vi "AOL Control.vi"() -> ()   [LabVIEW 2017]
uses:
  TypeDef/Frequency.ctl
  TypeDef/Amplitude.ctl
  TypeDef/AOL Mode.ctl
  Globals/FPGA Globals.vi
  <vilib>/DAQmx/create/channels.llb/DAQmx Create Channel (CO-Pulse Generation-Time).vi
panel:
  in  "DAQmx Digital Channel":tag="Dev1/ctr0"
  in  "Initial Delay(sec)":dbl=0.01 format="%.6f"
  in  "High Time(sec)":dbl=1e-05
  in  "Low Time(sec)":dbl=0.1
  in  "error in":errorcluster
  out "Select Device 2":i32=1 min=1 max=5 step=1
  out "Select Device 1":i32=1 min=1 max=5 step=1
  in  "Settings":bool
  in  "Refresh":bool
  in  "Save As":bool
  in  "Clear":bool
  in  "Run":bool
  in  "Load":bool
  in  "Stop":bool
  out "No of Packets":i32
  out "Packet Array":string[](array[string])
  in  "AOL Mode":T1=enum."Alignment"
  in  "Amplitude":T2={"Ch 1"=210, "Ch 2"=200, "Ch 3"=227, "Ch 4"=220, "Ch 5"=130, "Ch 6"=100, "Ch 7"=120, "Ch 8"=100}
  in  "Frequency (MHz)":T3={"Ch 1"=39, "Ch 2"=39, "Ch 3"=39, "Ch 4"=39, "Ch 5"=39, "Ch 6"=39, "Ch 7"=39, "Ch 8"=39}
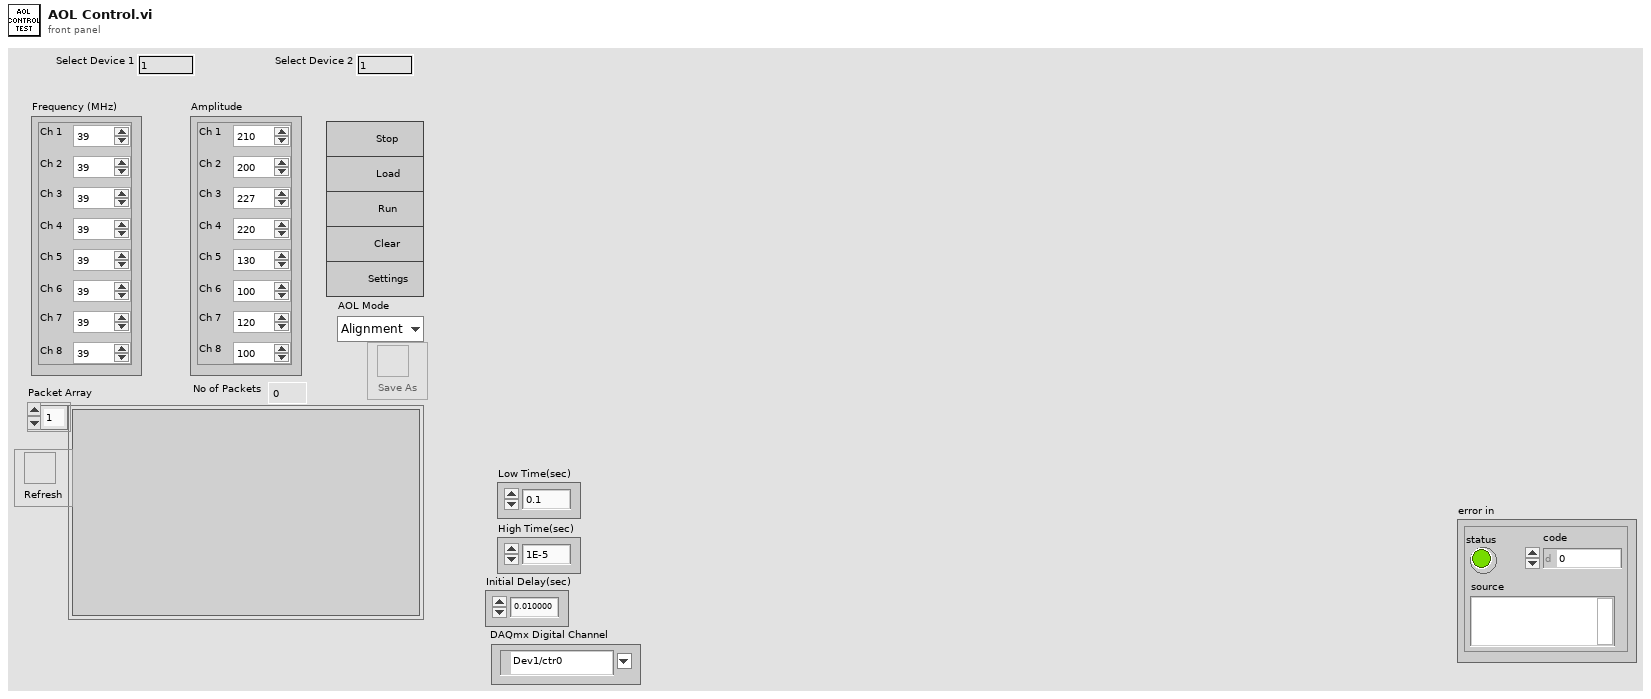
[diagram p1: front panel]
types:
  T1 = typedef "AOL Mode.ctl" = enum16{"Raster", "Structural", "Functional", "MiniScan", "Alignment"}
  T2 = typedef "Amplitude.ctl" = cluster{"Ch 1":u16, "Ch 2":u16, "Ch 3":u16, "Ch 4":u16, "Ch 5":u16, "Ch 6":u16, "Ch 7":u16, "Ch 8":u16}
  T3 = typedef "Frequency.ctl" = cluster{"Ch 1":u16, "Ch 2":u16, "Ch 3":u16, "Ch 4":u16, "Ch 5":u16, "Ch 6":u16, "Ch 7":u16, "Ch 8":u16}
  T4 = typedef "FPGA Settings.ctl" = cluster{"System Clock(MHz)":dbl, "FPGA MAC 1":string, "Port Number 1":i32, "Port Number 2":i32, "FPGA MAC 2":string}
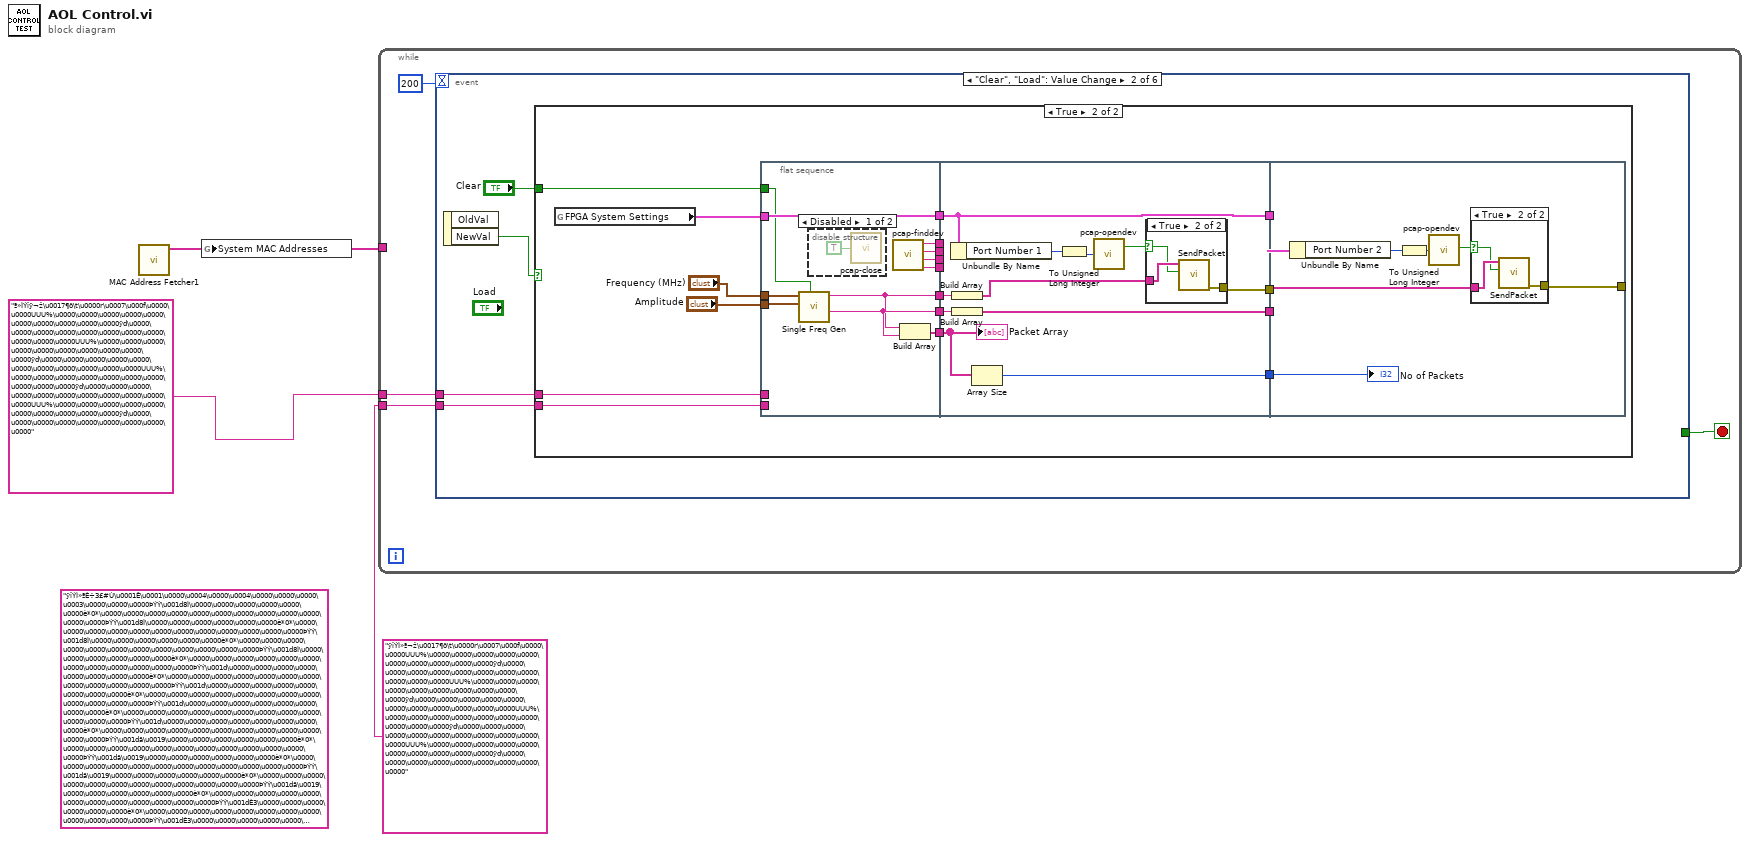
[diagram p0: block diagram]
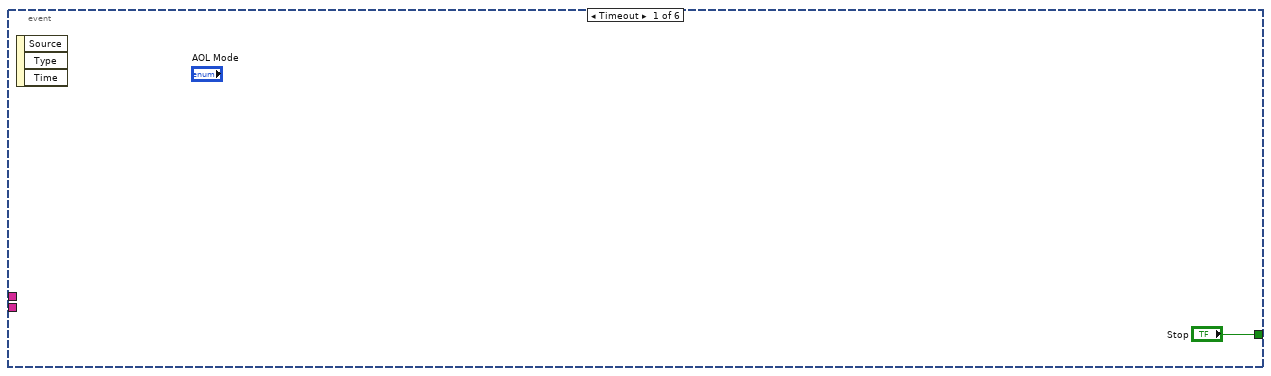
[diagram p2: hidden frame]
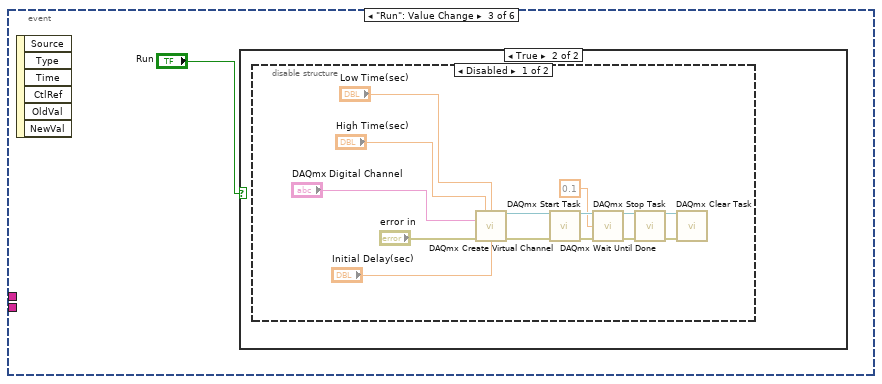
[diagram p7: hidden frame]
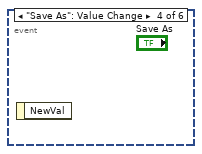
[diagram p10: hidden frame]
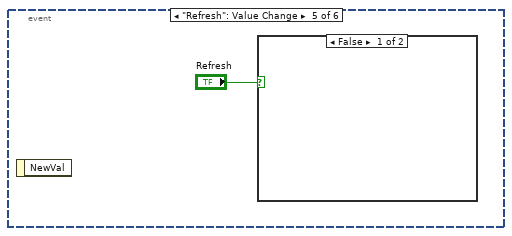
[diagram p11: hidden frame]
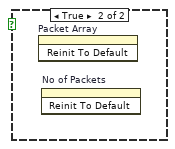
[diagram p12: hidden frame]
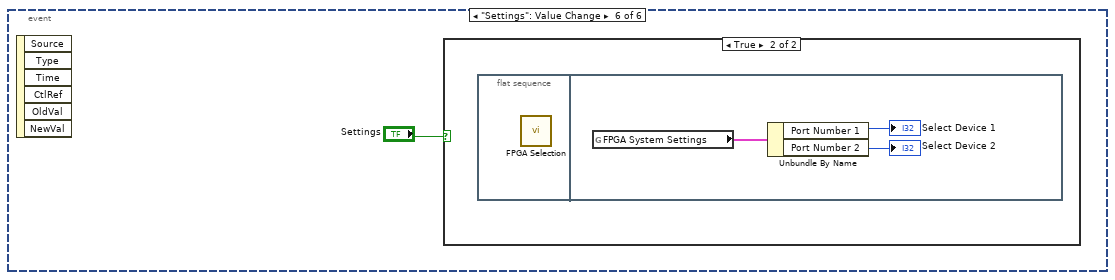
[diagram p13: hidden frame]
diagram:
  (unwired) "ÿîÝÌ»ªÈ÷3£#Ù\u0001Ê\u0001\u0000\u0004\u0000\u0004\u0000\u0000\u0000\u0003\u0000\u0000\u0000ÞÝÝ\u001d8Ì\u0000\u0000\u0000\u0000\u0000\u0000è*0*\u0000\u0000\u0000\u0000\u0000\u0000\u0000\u0000\u0000\u0000\u0000\u0000ÞÝÝ\u001d8Ì\u0000\u0000\u0000\u0000\u0000\u0000è*0*\u0000\u0000\u0000\u0000\u0000\u0000\u0000\u0000\u0000\u0000\u0000\u0000ÞÝÝ\u001d8Ì\u0000\u0000\u0000\u0000\u0000\u0000è*0*\u0000\u0000\u0000\u0000\u0000\u0000\u0000\u0000\u0000\u0000\u0000\u0000ÞÝÝ\u001d8Ì\u0000\u0000\u0000\u0000\u0000\u0000è*0*\u0000\u0000\u0000\u0000\u0000\u0000\u0000\u0000\u0000\u0000\u0000\u0000ÞÝÝ\u001d\u0000\u0000\u0000\u0000\u0000\u0000\u0000\u0000è*0*\u0000\u0000\u0000\u0000\u0000\u0000\u0000\u0000\u0000\u0000\u0000\u0000ÞÝÝ\u001d\u0000\u0000\u0000\u0000\u0000\u0000\u0000\u0000è*0*\u0000\u0000\u0000\u0000\u0000\u0000\u0000\u0000\u0000\u0000\u0000\u0000ÞÝÝ\u001d\u0000\u0000\u0000\u0000\u0000\u0000\u0000\u0000è*0*\u0000\u0000\u0000\u0000\u0000\u0000\u0000\u0000\u0000\u0000\u0000\u0000ÞÝÝ\u001d\u0000\u0000\u0000\u0000\u0000\u0000\u0000\u0000è*0*\u0000\u0000\u0000\u0000\u0000\u0000\u0000\u0000\u0000\u0000\u0000\u0000ÞÝÝ\u001dä\u0019\u0000\u0000\u0000\u0000\u0000\u0000è*0*\u0000\u0000\u0000\u0000\u0000\u0000\u0000\u0000\u0000\u0000\u0000\u0000ÞÝÝ\u001dä\u0019\u0000\u0000\u0000\u0000\u0000\u0000è*0*\u0000\u0000\u0000\u0000\u0000\u0000\u0000\u0000\u0000\u0000\u0000\u0000ÞÝÝ\u001dä\u0019\u0000\u0000\u0000\u0000\u0000\u0000è*0*\u0000\u0000\u0000\u0000\u0000\u0000\u0000\u0000\u0000\u0000\u0000\u0000ÞÝÝ\u001dä\u0019\u0000\u0000\u0000\u0000\u0000\u0000è*0*\u0000\u0000\u0000\u0000\u0000\u0000\u0000\u0000\u0000\u0000\u0000\u0000ÞÝÝ\u001dÈ3\u0000\u0000\u0000\u0000\u0000\u0000è*0*\u0000\u0000\u0000\u0000\u0000\u0000\u0000\u0000\u0000\u0000\u0000\u0000ÞÝÝ\u001dÈ3\u0000\u0000\u0000\u0000\u0000\u0000è*0*\u0000\u0000\u0000\u0000\u0000\u0000\u0000\u0000\u0000\u0000\u0000\u0000ÞÝÝ\u001dÈ3\u0000\u0000\u0000\u0000\u0000\u0000è*0*\u0000\u0000\u0000\u0000\u0000\u0000\u0000\u0000\u0000\u0000\u0000\u0000ÞÝÝ\u001dÈ3\u0000\u0000\u0000\u0000\u0000\u0000è*0*\u0000\u0000\u0000\u0000\u0000\u0000\u0000\u0000\u0000\u0000"
  n1 = call "MAC Address Fetcher1.vi"() -> ("MAC Addresses"=w3:string[])  [unwired: 9 in, 2 out]
  n2 = global write "FPGA Globals.vi" "System MAC Addresses"(w3) -> ()
  n3 = while {
    tunnel: w3 -> [_]
    tunnel: "ª»ÌÝîÿ¬ž\u0017¶ö\t\u0000r\u0007\u000f\u0000\u0000UUU%\u0000\u0000\u0000\u0000\u0000\u0000\u0000\u0000\u0000\u0000ÿd\u0000\u0000\u0000\u0000\u0000\u0000\u0000\u0000\u0000\u0000\u0000UUU%\u0000\u0000\u0000\u0000\u0000\u0000\u0000\u0000\u0000\u0000ÿd\u0000\u0000\u0000\u0000\u0000\u0000\u0000\u0000\u0000\u0000\u0000UUU%\u0000\u0000\u0000\u0000\u0000\u0000\u0000\u0000\u0000\u0000ÿd\u0000\u0000\u0000\u0000\u0000\u0000\u0000\u0000\u0000\u0000\u0000UUU%\u0000\u0000\u0000\u0000\u0000\u0000\u0000\u0000\u0000\u0000ÿd\u0000\u0000\u0000\u0000\u0000\u0000\u0000\u0000\u0000" ("String") -> [w5]
    tunnel: "ÿîÝÌ»ª¬ž\u0017¶ö\t\u0000r\u0007\u000f\u0000\u0000UUU%\u0000\u0000\u0000\u0000\u0000\u0000\u0000\u0000\u0000\u0000ÿd\u0000\u0000\u0000\u0000\u0000\u0000\u0000\u0000\u0000\u0000\u0000UUU%\u0000\u0000\u0000\u0000\u0000\u0000\u0000\u0000\u0000\u0000ÿd\u0000\u0000\u0000\u0000\u0000\u0000\u0000\u0000\u0000\u0000\u0000UUU%\u0000\u0000\u0000\u0000\u0000\u0000\u0000\u0000\u0000\u0000ÿd\u0000\u0000\u0000\u0000\u0000\u0000\u0000\u0000\u0000\u0000\u0000UUU%\u0000\u0000\u0000\u0000\u0000\u0000\u0000\u0000\u0000\u0000ÿd\u0000\u0000\u0000\u0000\u0000\u0000\u0000\u0000\u0000" ("String") -> [w4]
    stop <- w6 stop-if-true
    n4 = event shown="[1] \"Clear\", \"Load\": Value Change" {
      selector: _ -> [_ _ _ _ _ _]
      dyn-events: _ -> [_ _ _ _ _ _]
      timeout: 200 -> [_ _ _ _ _ _]
      tunnel: ["Stop" _ _ _ _ _] -> w6
      tunnel: w5 -> [_ w10 _ _ _ _]
      tunnel: w4 -> [_ w9 _ _ _ _]
      event Timeout {
        n5 = event-data() -> ()  [unwired: 1 in, 3 out]
      }
      event "Clear", "Load": Value Change {
        n6 = event-data() -> ("NewVal"=w12:bool)  [unwired: 1 in, 1 out]
        n7 = case shown="True" w12 {
          tunnel: "Clear" -> [_ w21]
          tunnel: w10 -> [_ w16]
          tunnel: w9 -> [_ w15]
          frame False {
          }
          frame True {
            n8 = global read "FPGA Globals.vi" "FPGA System Settings"() -> (w22:T4)
            n9 = flat-sequence {
              tunnel: "Amplitude" -> [w41]
              tunnel: "Frequency (MHz)" -> [w40]
              tunnel: [w39] -> w30
              tunnel: [w38] -> w29
              tunnel: w22 -> [w38]
              tunnel: w21 -> [w37]
              tunnel: [w36] -> w20
              tunnel: [w35] -> w19
              tunnel: [w34] -> w18
              tunnel: [w33] -> w17
              tunnel: w16 -> [_]
              tunnel: w15 -> [_]
              tunnel: [w31] -> w14
              tunnel: [w32] -> w13
              tunnel: [w52] -> w28
              tunnel: [w48] -> w27
              tunnel: w30 -> [w47]
              tunnel: [w46] -> w26
              tunnel: w29 -> [w43]
              tunnel: [w43] -> w25
              tunnel: w20 -> [_]
              tunnel: w19 -> [_]
              tunnel: w18 -> [_]
              tunnel: w17 -> [_]
              tunnel: w14 -> [w51]
              tunnel: w13 -> [w50]
              tunnel: w28 -> [_]
              tunnel: [w62] -> _
              tunnel: w27 -> [w61]
              tunnel: w26 -> [w60]
              tunnel: w25 -> [w59]
              frame #0 {
                n10 = call "Single Freq Gen.vi"("Stop Single Frquency"=w37, "Amplitude"=w41, "Frequency (MHz)"=w40) -> ("Hex String 2"=w32:string, "Hex String 1"=w31:string)  [unwired: 7 in]
                n11 = disable-structure shown="Disabled" {
                  frame Disabled {
                    n12 = call "pcap-close.vi"("Opened"=TRUE) -> ()
                  }
                  frame Enabled {
                  }
                }
                n13 = call "pcap-finddev.vi"() -> ("String 4"=w33:string, "String 3"=w34:string, "String 2"=w35:string, "String"=w36:string)  [unwired: 1 in, 1 out]
                n14 = Build Array(w31, w32) -> (w39:string[])
              }
              frame #1 {
                n15 = Unbundle By Name(w43) -> ("Port Number 1"=w45:i32)
                n16 = Build Array(w51) -> (w49:string[])
                n17 = Build Array(w50) -> (w48:string[])
                n18 = Array Size(array=w47) -> (size(s)=w46:i32)
                n19 = To Unsigned Long Integer(number=w45) -> (unsigned 32bit integer=w44:u32)
                n20 = call "pcap-opendev.vi"("Select Device"=w44) -> ("Opened"=w53:bool)  [unwired: 2 out]
                n21 = case shown="True" w53 {
                  selector: w53 -> [_ w54]
                  tunnel: [_ w56] -> w52
                  tunnel: w49 -> [_ w55]
                  frame False {
                  }
                  frame True {
                    n22 = call "SendPacket.vi"("Ethernet Port Opened ?"=w54, "Packet Array"=w55) -> ("error out"=w56:errorcluster)  [unwired: 8 in, 1 out]
                  }
                }
                "Packet Array" <- w47
              }
              frame #2 {
                n23 = Unbundle By Name(w59) -> ("Port Number 2"=w58:i32)
                n24 = To Unsigned Long Integer(number=w58) -> (unsigned 32bit integer=w57:u32)
                n25 = call "pcap-opendev.vi"("Select Device"=w57) -> ("Opened"=w63:bool)  [unwired: 2 out]
                n26 = case shown="True" w63 {
                  selector: w63 -> [_ w64]
                  tunnel: [_ w66] -> w62
                  tunnel: w61 -> [_ w65]
                  frame False {
                  }
                  frame True {
                    n27 = call "SendPacket.vi"("Ethernet Port Opened ?"=w64, "Packet Array"=w65) -> ("error out"=w66:errorcluster)  [unwired: 8 in, 1 out]
                  }
                }
                "No of Packets" <- w60
              }
            }
          }
        }
      }
      event "Run": Value Change {
        n28 = event-data() -> ()  [unwired: 1 in, 6 out]
        n29 = case shown="True" "Run" {
          frame False {
          }
          frame True {
            n30 = disable-structure shown="Disabled" {
              frame Disabled {
                n31 = call-poly <vilib>:"DAQmx Create Virtual Channel.vi"("high time"="High Time(sec)", "low time"="Low Time(sec)", "counter"="DAQmx Digital Channel", "error in"="error in", "initial delay"="Initial Delay(sec)") -> ("task out"=w76:refnum<k21>, "error out"=w75:errorcluster)  [unwired: 9 in]
                n32 = call <vilib>:"DAQmx Start Task.vi"("task/channels in"=w76, "error in"=w75) -> ("task out"=w74:refnum<k21>, "error out"=w70:errorcluster)  [unwired: 12 in]
                n33 = call <vilib>:"DAQmx Wait Until Done.vi"("task/channels in"=w74, "timeout (sec)"=0.1, "error in"=w70) -> ("task out"=w69:refnum<k21>, "error out"=w68:errorcluster)  [unwired: 11 in]
                n34 = call <vilib>:"DAQmx Stop Task.vi"("task/channels in"=w69, "error in"=w68) -> ("task out"=w73:refnum<k21>, "error out"=w72:errorcluster)  [unwired: 12 in]
                n35 = call <vilib>:"DAQmx Clear Task.vi"("task in"=w73, "error in"=w72) -> ()  [unwired: 13 in, 1 out]
              }
              frame Enabled {
              }
            }
          }
        }
      }
      event "Save As": Value Change {
        n36 = event-data() -> ()  [unwired: 1 in, 1 out]
      }
      event "Refresh": Value Change {
        n37 = event-data() -> ()  [unwired: 1 in, 1 out]
        n38 = case shown="False" "Refresh" {
          frame False {
          }
          frame True {
            n39 = invoke on="Packet Array" class="Arr (strict)" method="Reinit To Default"() -> ()  [unwired: 3 in, 3 out]
            n40 = invoke on="No of Packets" class="DigNum (strict)" method="Reinit To Default"() -> ()  [unwired: 3 in, 3 out]
          }
        }
      }
      event "Settings": Value Change {
        n41 = event-data() -> ()  [unwired: 1 in, 6 out]
        n42 = case shown="True" "Settings" {
          frame False {
          }
          frame True {
            n43 = flat-sequence {
              frame #0 {
                n44 = call "FPGA Selection.vi"() -> ()  [unwired: 12 in]
              }
              frame #1 {
                n45 = global read "FPGA Globals.vi" "FPGA System Settings"() -> (w84:T4)
                n46 = Unbundle By Name(w84) -> ("Port Number 1"=→"Select Device 1":i32, "Port Number 2"=→"Select Device 2":i32)
              }
            }
          }
        }
      }
    }
  }
